vi "pwm testing.vi"() -> ()   [LabVIEW 2015]
uses:
  <vilib>/myRIO/Instrument Drivers/Onboard IO/PWM/typedefs/PWM Reference.ctl
  <vilib>/myRIO/Common/Instrument Driver Framework/Utilities/typedefs/myRIO Generic Hardware Reference.ctl
  <vilib>/myRIO/Common/Instrument Driver Framework/Utilities/typedefs/Hardware Version Enum.ctl
  <vilib>/myRIO/Common/Instrument Driver Framework/Utilities/typedefs/myRIO v1.0 Reference.ctl
  <vilib>/myRIO/Common/Instrument Driver Framework/Utilities/typedefs/Generic FPGA Reference.ctl
  <vilib>/myRIO/Common/Instrument Driver Framework/myRIO v1.0/PWM/typedefs/PWM Channels Enum.ctl
  <vilib>/myRIO/Instrument Drivers/Onboard IO/PWM/typedefs/PWM Configuration.ctl
  <vilib>/userdefined/High Color/nirio_resource_hc.ctl
  <vilib>/myRIO/Common/Instrument Driver Framework/myRIO v1.0/PWM/vis/myRIO v1.1 Open PWM.vi
  <vilib>/myRIO/Common/Instrument Driver Framework/Utilities/vis/Validate Channels.vi
  <vilib>/myRIO/Common/Instrument Driver Framework/myRIO v1.0/PWM/vis/myRIO v1.0 Reserve PWM.vi
  <vilib>/myRIO/Common/Instrument Driver Framework/myRIO v1.0/PWM/vis/myRIO v1.0 Build MUX Configuration PWM.vi
  <vilib>/myRIO/Common/Instrument Driver Framework/myRIO v1.0/Resource Manager/vis/myRIO v1.0 Reserve Channel List.vi
  <vilib>/myRIO/Common/Instrument Driver Framework/myRIO v1.0/Resource Manager/vis/myRIO v1.0 Create Configuration List.vi
  <vilib>/myRIO/Common/Instrument Driver Framework/myRIO v1.0/Resource Manager/vis/myRIO v1.0 Reserve Channel.vi
  <vilib>/myRIO/Common/Instrument Driver Framework/myRIO v1.0/Resource Manager/vis/myRIO v1.0 Unreserve Channel.vi
  <vilib>/myRIO/Common/Instrument Driver Framework/myRIO v1.0/Resource Manager/vis/myRIO v1.0 Build Mutex Name.vi
  <vilib>/Utility/VariantDataType/GetNumericInfo.vi
  <vilib>/Utility/error.llb/Error Cluster From Error Code.vi
  <vilib>/myRIO/Common/Instrument Driver Framework/myRIO v1.0/myRIO v1.1 Open.vi
  <vilib>/myRIO/Common/Instrument Driver Framework/Utilities/vis/IO Manager.vi
  <vilib>/myRIO/Common/Instrument Driver Framework/Utilities/vis/Configuration Manager.vi
  <vilib>/myRIO/Common/Instrument Driver Framework/myRIO v1.0/Resource Manager/vis/myRIO v1.0 Configure IO.vi
  <vilib>/myRIO/Common/Instrument Driver Framework/myRIO v1.0/myRIO v1.0 Close.vi
  <vilib>/myRIO/Common/Instrument Driver Framework/myRIO v1.0/PWM/vis/myRIO v1.0 Write PWM.vi
  <vilib>/addons/control/pid/pid.llb/PID (DBL).vi
  <vilib>/myRIO/Instrument Drivers/Onboard IO/PWM/vis/myRIO PWM Open.xnode
  <vilib>/myRIO/Instrument Drivers/Onboard IO/PWM/PWM.lvlib
  <vilib>/addons/control/pid/NI_PID_pid.lvlib
panel:
  in  "set point":dbl min=-0.13333 max=0.1333 step=0.005
  out "Elapsed Time (s)":dbl
  out ".not. x? 2":bool
  out "feedback":dbl
  out "desired pwm":dbl
  in  "PID gains 2":T1={"proportional gain (Kc)"=0.002, "integral time (Ti, min)"=7e-07, "derivative time (Td, min)"=0.0} {"derivative time (Td, min)" format="%.8f"; "integral time (Ti, min)" format="%.8f"; "proportional gain (Kc)" format="%.8f"}
  in  "output range 2":cluster{"output high":dbl, "output low":dbl}={"output high"=0.25, "output low"=-0.25} {"output low" format="%.6f"; "output high" format="%.5f"}
  out "dt out (s) 2":dbl format="%.3f"
  out "Waveform Chart":dbl(graph)
  in  "stop 2":bool
  out "actual pwm":dbl
  in  "Allow multiple opens?":bool=TRUE
  in  "stop":bool
  in  "Duty Cycle":dbl=0.5 min=0.05 max=0.1 step=0.001
  in  "Frequency [Hz]":dbl=333.33
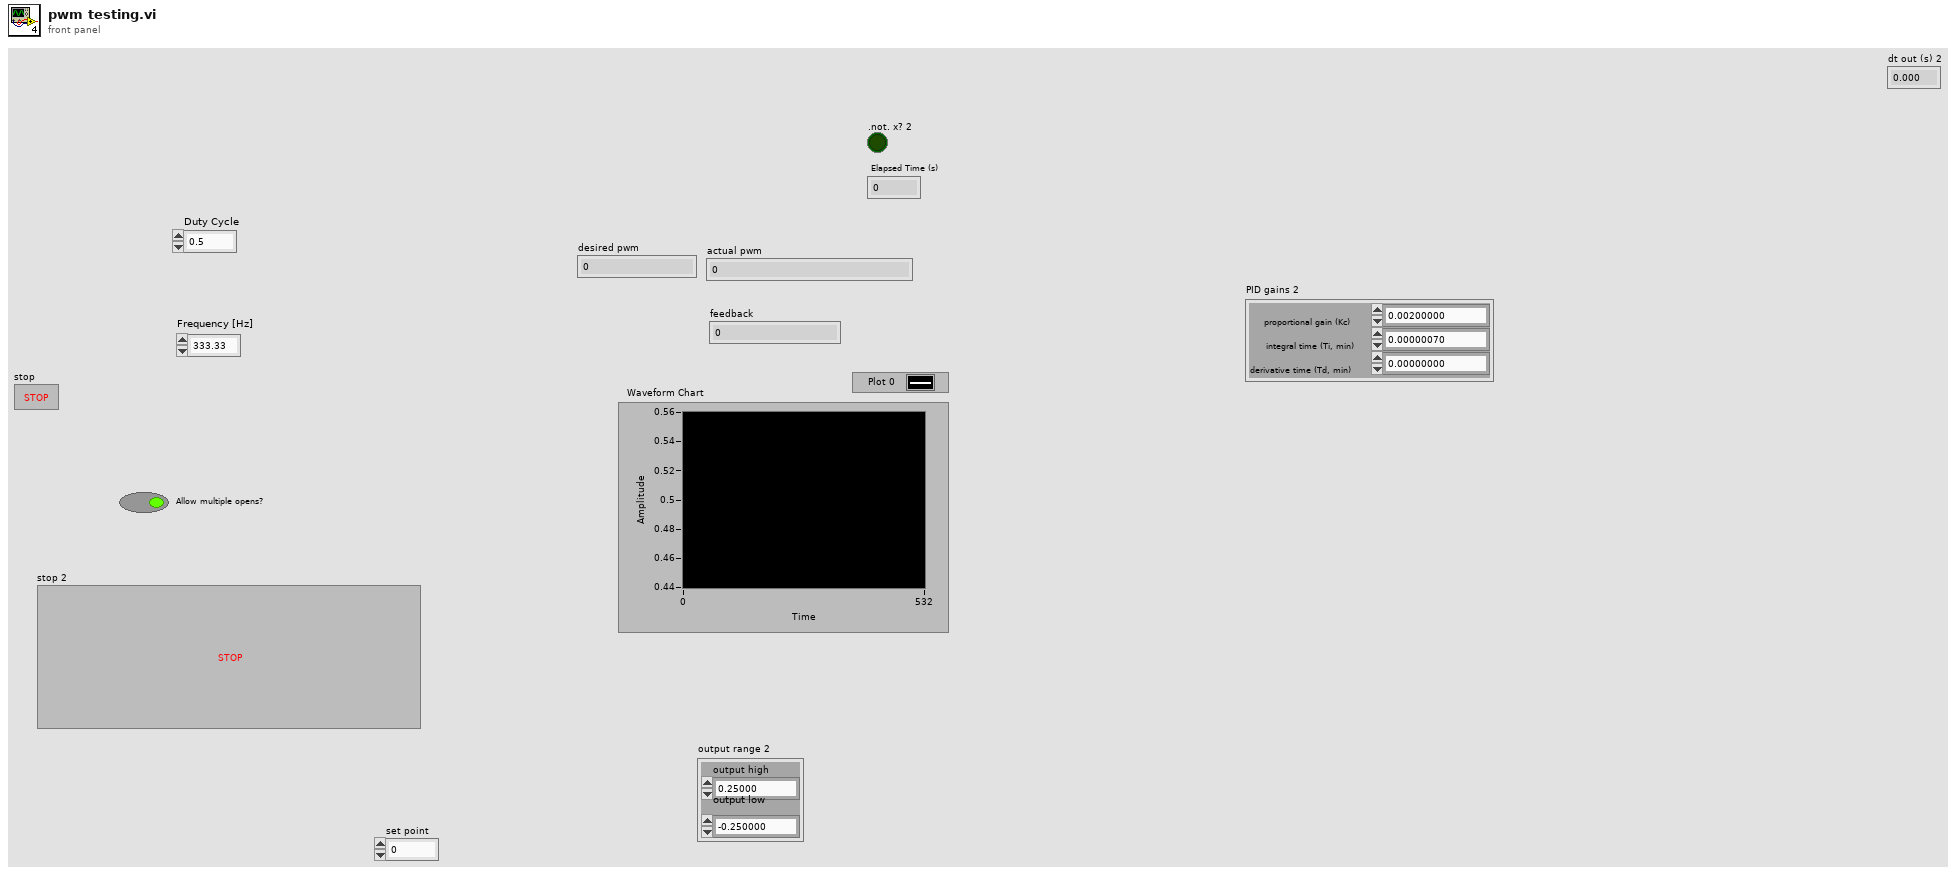
[diagram p1: front panel]
types:
  T1 = cluster{"proportional gain (Kc)":dbl, "integral time (Ti, min)":dbl, "derivative time (Td, min)":dbl}
  T2 = typedef "nirio_resource_hc.ctl" = tag
  T3 = typedef "Hardware Version Enum.ctl" = enum16{"Unknown", "myRIO-1900", "myRIO-1950", "roboRIO"}
  T4 = typedef "PWM.lvlib/PWM Reference.ctl" = cluster{"myRIO Reference":T5, "PWM Channels Enum":T8, "PWM Configuration":T9}
  T5 = typedef "myRIO Generic Hardware Reference.ctl" = cluster{"myRIO Model":T3, "myRIO Hardware Reference":T6}
  T6 = typedef "myRIO v1.0 Reference.ctl" = cluster{"Generic FPGA Reference":T7, "Allow multiple opens":bool}
  T7 = typedef "Generic FPGA Reference.ctl" = refnum<k20>
  T8 = typedef "PWM Channels Enum.ctl" = enum16{"Not Connected", "C/PWM0", "C/PWM1", "A/PWM0", "A/PWM1", "A/PWM2", "B/PWM0", "B/PWM1", "B/PWM2", "PWM/PWM0", "PWM/PWM1", "PWM/PWM2", "PWM/PWM3", "PWM/PWM4", "PWM/PWM5", "PWM/PWM6", "PWM/PWM7", "PWM/PWM8", "PWM/PWM9"}
  T9 = typedef "PWM.lvlib/PWM Configuration.ctl" = cluster{"Frequency":dbl, "Duty Cycle":dbl}
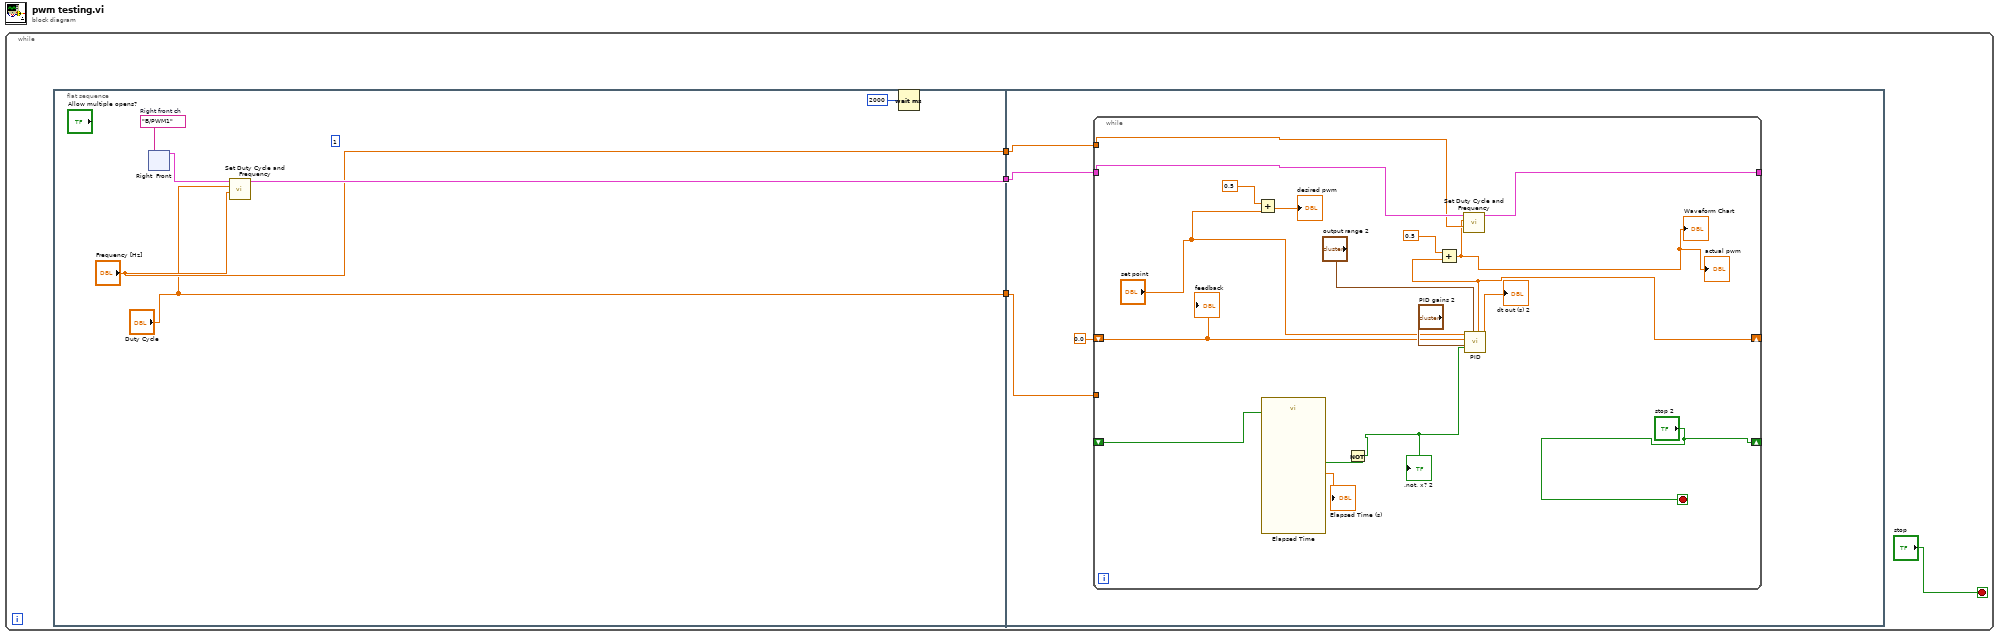
[diagram p0: block diagram]
diagram:
  n1 = while {
    stop <- "stop" stop-if-true
    n2 = flat-sequence {
      tunnel: [w9] -> w4
      tunnel: ["Frequency [Hz]"] -> w2
      tunnel: ["Duty Cycle"] -> w1
      tunnel: w4 -> [w30]
      tunnel: w2 -> [w29]
      tunnel: w1 -> [w28]
      frame #0 {
        w7 = tag "B/PWM1"  # Right front ch
        (unwired) 1
        n3 = xnode "Right  Front"("Channel Name"=w7) -> ("PWM Ref Out"=w6:T4)  [unwired: 2 in, 1 out]
        n4 = call <vilib>:"Set Duty Cycle and Frequency.vi"("Frequency [Hz]"="Frequency [Hz]", "Duty Cycle"="Duty Cycle", "PWM Ref In"=w6) -> ("PWM Ref Out"=w9:T4)  [unwired: 6 in, 1 out]
        n5 = Wait (ms)(milliseconds to wait=u32 2000) -> ()  [unwired: 1 out]
      }
      frame #1 {
        n6 = while {
          tunnel: w30 -> [w47]
          tunnel: [w48] -> _
          tunnel: w29 -> [w46]
          tunnel: w28 -> [_]
          shift-right: [w32] -> _
          shift-left: 0.0 ("output") -> [w42]
          shift-right: ["stop 2"] -> _
          shift-left: _ -> [w36]
          stop <- "stop 2" stop-if-true
          n7 = Add(x=0.5, y="set point") -> (x+y=→"desired pwm":dbl)
          n8 = call "Elapsed Time"("Reset"=w36) -> ("Elapsed Time (s)"=→"Elapsed Time (s)":dbl, "Time has Elapsed"=w39:bool)  [unwired: 11 in, 6 out]
          n9 = Not(x=w39) -> (.not. x?=w38:bool)
          ".not. x? 2" <- w38
          n10 = call-poly <vilib>:"PID.vi"("reinitialize? (F)"=w38, "output range"="output range 2", "PID gains"="PID gains 2", "process variable"=w42, "setpoint"="set point") -> ("dt out (s)"=→"dt out (s) 2":dbl, "output"=w32:dbl)  [unwired: 5 in]
          n11 = Add(x=0.5, y=w32) -> (x+y=w40:dbl)
          "actual pwm" <- w40
          "Waveform Chart" <- w40
          n12 = call <vilib>:"Set Duty Cycle and Frequency.vi"("Frequency [Hz]"=w46, "Duty Cycle"=w40, "PWM Ref In"=w47) -> ("PWM Ref Out"=w48:T4)  [unwired: 6 in, 1 out]
          "feedback" <- w42
        }
      }
    }
  }
